vi "_RSA_PKCS1.vi"() -> ()   [LabVIEW 2023]
uses:
  <vilib>/addons/Tools/Unicode/UTF8 Tools.lvlib
panel:
  out "tick":u32
  in  "Tab Control":enum32{"密钥生成", "加密解密"}(tab)
  in  "生成秘钥":bool
  in  "填入密钥":bool
  out "公钥":string
  out "私钥":string
  out "?":string
  in  "密钥位数":string(combo)="308"
  in  "原文":string="Lorem ipsum dolor sit amet, consectetur adipisicing elit, sed do eiusmod tempor incididunt ut labore et dolore magna aliqua. Ut enim ad minim veniam, quis nostrud exercitation ullamco laboris nisi ut aliquip ex ea commodo consequat. Duis aute irure dolor in reprehenderit in voluptate velit esse cillum dolore eu fugiat nulla pariatur. Excepteur sint occaecat cupidatat non proident, sunt in culpa qui officia deserunt mollit anim id est laborum.\n"
  out "密文":string
  in  "密文":string="HCpIgJk/+R0CBhNWtByPKFZV9ITOXw7kY+R+gOsu/5SOpf9Kbk8F4EOCOOqLRaOCJf+GX3E+qD7oYj5SvAQCmhEU2YjpwG/wUmATbHKIMHQXZ3Rc/3We3BmbNaJrOw91EL7mVTCTQKMjuYVXiq0hajnJ+BwQXjJZfybkTRK94pGxM9G/5ZSGuP/ewRceAxQ0yhsyaCqbmHTiLNz3D6rYzJVMYsk9he5zXvHd+kh1cd+ASKWMB/Vgven+oDARy3ejDRk9U+cizFmNVrMUm57ClIMOirlQBShpa4uk4ZT/V0xm4sjeT+4QGanPMXhPoeHUftwo90kfVObeDCtFEM2rLgbRJHz2MoithAR2BuClGDqlx9vAYB7Ei8+WXeRKjW2AGi5rbdkcxlkdCeyQ6jcfV9paWfaTqELMHz1mj0miOK4jqfBWrivbPosi/fbzTefCRTtqdfDHCHDBJEmWznu712J68iJhvN7u1yrtBICKOHmNUei+4WFPm9bCTvQTIsQwz9hw1AqzWC64baBmIqTIvQTLyRJGjv1r6ERQIzWghyR0TXT+WTQWQxtIw4FetOOwLbTf1QXrQ6BoldZv3V28DkhC6P5vZM3x5ITuw08wj6Mt+oF41Nz+4hs4VaUNOiR2nf6cN2cOJvifRCPmeqlWFlGcHpX0+CvA145GZyN4+98="
  out "原文":string
  in  "加密":bool
  in  "解密":bool
  in  "公钥":string="-----BEGIN RSA PUBLIC KEY-----\nMIICCQKCAgBD33IPuq3zWwZXK/81Ebsg/7gVrV2vQ5o/0i/0ae8N/OOdEqVAupkM\nojXLqbPXJel1KlvTVMRJNtU45WlqnPDlWNInK6aqiPJHPAjOrX/lrrnaPksvRA2r\nfRN8VgmVZeQdT85luT3FWqZP7G2fsZq5Tp2bcm7265mnbctFlmg7BziyM5KmA5Hy\noUOkXDm2nWWwvsrr9evwZDpZTrLF2RoEP3Kb4uRrzjIEhBZer7fuM/m/wE728WyT\nuenw88mhmYYKpUHQn67jfuxqHOeFkRH/ShbL569eOh3pl2tDGEa7UTFxu31HLwje\n0zU3s59TWHqb7uISH5Dk+EqhKb3JfnHh5DfCO8qg7fRxGCk7yR6wb7WOG7kLnXz0\nuDfnWafYPiBqjywEnYkp8haQVAZSHtmvHw+ssjSRFV1kE0oMMB35+VKw1jkcQIQT\nxs9diDMW0j5Hb+LM86E5JwR3tKEHr3HWgOBcZJZ0woZGJ+gmNJ42F7XYxaeobkSR\nSRrFbEucK+l4q4FpkgwVS8L9NbUsu2CclK+Z2OI44Q3p44VI7ph6nfZrrVR02sHo\n5rIES8rVwXDdT1ory/Dq3SCOIRL6QC5zh6NTgZSYzwH1Jh8ufi07N+JToR1gdpM5\nc5wTTrmpFF+Ujk8lPEx7yZcZDbm70+2b9mAL7h+/7wy6Ia2Zjx4kGQIDAQAB\n-----END RSA PUBLIC KEY-----"
  in  "私钥":string="-----BEGIN RSA PRIVATE KEY-----\nMIIJJQIBAAKCAgBD33IPuq3zWwZXK/81Ebsg/7gVrV2vQ5o/0i/0ae8N/OOdEqVA\nupkMojXLqbPXJel1KlvTVMRJNtU45WlqnPDlWNInK6aqiPJHPAjOrX/lrrnaPksv\nRA2rfRN8VgmVZeQdT85luT3FWqZP7G2fsZq5Tp2bcm7265mnbctFlmg7BziyM5Km\nA5HyoUOkXDm2nWWwvsrr9evwZDpZTrLF2RoEP3Kb4uRrzjIEhBZer7fuM/m/wE72\n8WyTuenw88mhmYYKpUHQn67jfuxqHOeFkRH/ShbL569eOh3pl2tDGEa7UTFxu31H\nLwje0zU3s59TWHqb7uISH5Dk+EqhKb3JfnHh5DfCO8qg7fRxGCk7yR6wb7WOG7kL\nnXz0uDfnWafYPiBqjywEnYkp8haQVAZSHtmvHw+ssjSRFV1kE0oMMB35+VKw1jkc\nQIQTxs9diDMW0j5Hb+LM86E5JwR3tKEHr3HWgOBcZJZ0woZGJ+gmNJ42F7XYxaeo\nbkSRSRrFbEucK+l4q4FpkgwVS8L9NbUsu2CclK+Z2OI44Q3p44VI7ph6nfZrrVR0\n2sHo5rIES8rVwXDdT1ory/Dq3SCOIRL6QC5zh6NTgZSYzwH1Jh8ufi07N+JToR1g\ndpM5c5wTTrmpFF+Ujk8lPEx7yZcZDbm70+2b9mAL7h+/7wy6Ia2Zjx4kGQIDAQAB\nAoICADB+cPeOEQVELxaPh+t5/LLKItPSJ5K3AXnCCqNeIQBkhJhQnyPNbtbY+wjF\n+ompO9GL70niUdBhzhy1xQj4kyG6wYRdKtrDuB9vZHeO/Ue0/HNTeNKPlBjH5+k5\na+WDhGXxBG4n2VutthB6w6SK+BqYcgGD1Ia1tPYse0T//v7V3Qttz8Sv3lJ2KGdB\nwbaZZPPQjhnjfq0mX445rX+w62bHknKQvVXNYG1blsQWVptqJXJ8y66itkoiVmTj\nOlgs4dmvU4Pk48cFg5MZjc4f5bT6Ualkoyb27TJeDrREnxztGR/CrvLyRys1yts+\nioK5P/kzx/Dc/uCqCmB1+3UA1Ao/ptmaV1ZDMoYMTlaXkqPap6WsDN/I8p7xmSw9\n2LtirL6zHXTw5lIfoW87+lCdM37QtRexYCZPZH0kaGTs+xGVBiCdAsPyPqkoiFpP\noKkx0GRHmaZ0zab2Id6l+SBifzEa/6IU/t94mbsDyK/eK9AZjZhLjLreZEZmQWci\n8/c9NKOItkxBf+mLdxZDqeCmYHV4PbojLpCxqD0ngNo/y5CkegvP/Maq+6zkQ/Ci\nSIjUFnALqJx+HXf1BE+Qbs5TGOWLrs1y4+w8S4OnJ6S7ueVI/DkLlDHcT5c5S+W8\n/3/T1C/vgiJCKcT46sQAsl4KKIy6vKpQxtoMMbxe7zxVDgqRAoIBAQFz+6P3Y0to\nWhyAtUCneU6J/CN/ysVUr9EvvO/2fFYDSTeM3b7O1wvbkTanDFON/kbaDLllMp5S\nfWmkyWXcgm8lQ/Y7qakM902OPZ0hHLRrVyA2UcommOxhFCi5UrLJVtNkvxn44jpy\n1J2b7Pwap+pispIXdFEJ4So0It7Oh7V/XcOP0t7n4zM1EZ1qjnX6YCi3JinrB/9t\nQhlDLypv8ONLHx1EjBsVj21fMg1hAk32Clv4eS+EcNq6iqkJSmBFpsrGEkppLy8L\npmu4Og0S1D632tEXDDNTOc8RqD1aHkAVMYnnCPTWgd8W2DrAVXOjUL9HZXH84exV\nFfBYZQdFdiylAoIBAC611+BcPkzHP1B4giNZux1KMM5xwsGczd9Uwdjqm1JoquNn\njA2VSJhvIIOkSxkN8hh/lUpUXhWM7HJ8M/1eWcgrBJyskBnKb64fHIetZ6Ry9urD\nW5XO2MRAEfgN42F1P/glfv5UAjL+5/PBR69ddEV9YW42dJNAhfaIouzkFdEBxbXC\nJEE+bzoW3NcFCNCOJV0u41HQ0lLwWPqTz9zIqkGT0tAb26exyqfo/qmyIBnTT+Cd\ncXr8GKDgJZGOpTg7K4hy/L2+OJiAd8Lem9wkiMb8IfDqAdR0o50QFDXu1D/10CgK\nvCMBIUMlUWkzf/q8b39H/SAPt6tfZjsiRcG6u2UCggEAQDS/KIRLD8f+A3lFn6Kg\nm9CZkAU/6k4unT7PbIwpjIemvvnHZYxYz51RAaRvB6NMN3bayUzjZvmesoLQwi8B\nYD1K0yGFvGczS8n2xTBfM+fl93pGmkLrChagsNxFX9tMwab6pKrny8pHKhLNsQwq\nuL552PKKylnDHxyluKBUA5f7mWeccgoVXKOduDa+xmiynmpH8fl/bSxrj90kRg4e\nLWlBdAN66U3IYxYQmR38tusy1MCWIxYXqvskEiZ0V5Fijq25ik5KoIgpL7NVblqU\nOMfcL047zbG8vB9994AhL4dNdkNlf2ELULYh7fDR9O6LFZe9BRk54bXXtmo5xxOO\nwQKCAQAihZrK4uHYdNnCa44i+kpkV1TC/yjlVzKAgG/UFXA988V41CqaT16b6mWp\nZV9rYPcwS/rWOIxgeQq3gjwaYgUQ/1olQRQvO4JWuf+n9uzGiYEb+M5TZdCnGoMt\nRXZrrPBeQbgd15DYh7R+XrbQUM2CHixH/E8kFWfs0Qc49Ul6c0jgEGAjKDWkRQlq\nkPn2yVesCt9OtHr9eU0JxPy3PEc4uDvyOuSYh7ozZuvwFwnKjHZYl4QrVO4O2Bpr\n/XT2niSKcBGDWncRnsDkcQnYJdhA2E9tckVv89SIXD3TrnOH4fC551UsucUPjyEg\nE0Pe2C2/cEEP1Q31xkgUJDxR9eRRAoIBAGHW55fOf4K0b9SMA4+qDjSTC8FR8wjk\npKOPGwTb0qDzi1GgoFkViyBNeXbi/XhGvSgxktHB5rLHua5RV2CZ4hskDZFzHo12\nLTsHepyafJDLLefxP3ZXSOxKygcnBthiVShdR+Psk1xfljAWSxNTvHzhxIuzYCIq\nHgDA9mN/Ox47I3IktFOWXFYLp886eG4WXVYBW8DJ1ylreMCVZp2/R+ut25bnVfXS\n2DHVDJ325mwEP9aRwGh+KpbcA81X6KkZYtDIHzKOYRyp3exx05dFTQCceyXBOCHm\noG/bIfyOu/fk8RTQh3IRaIlvUEtZq5R5FmaHW/MMpnYutrLj1o00RUQ=\n-----END RSA PRIVATE KEY-----"
  in  "填入密文":bool
  out "加解密提示":string
  in  "填入密钥":bool
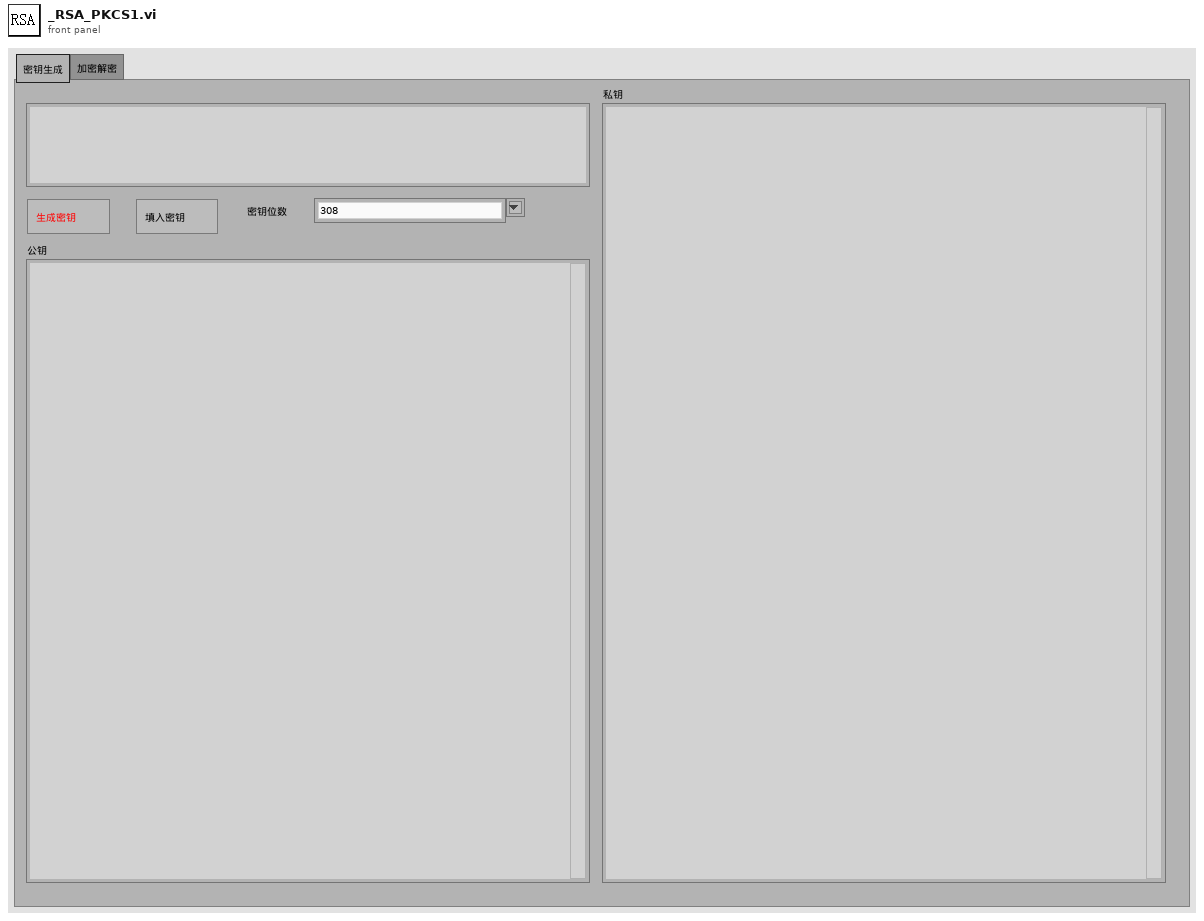
[diagram p1: front panel]
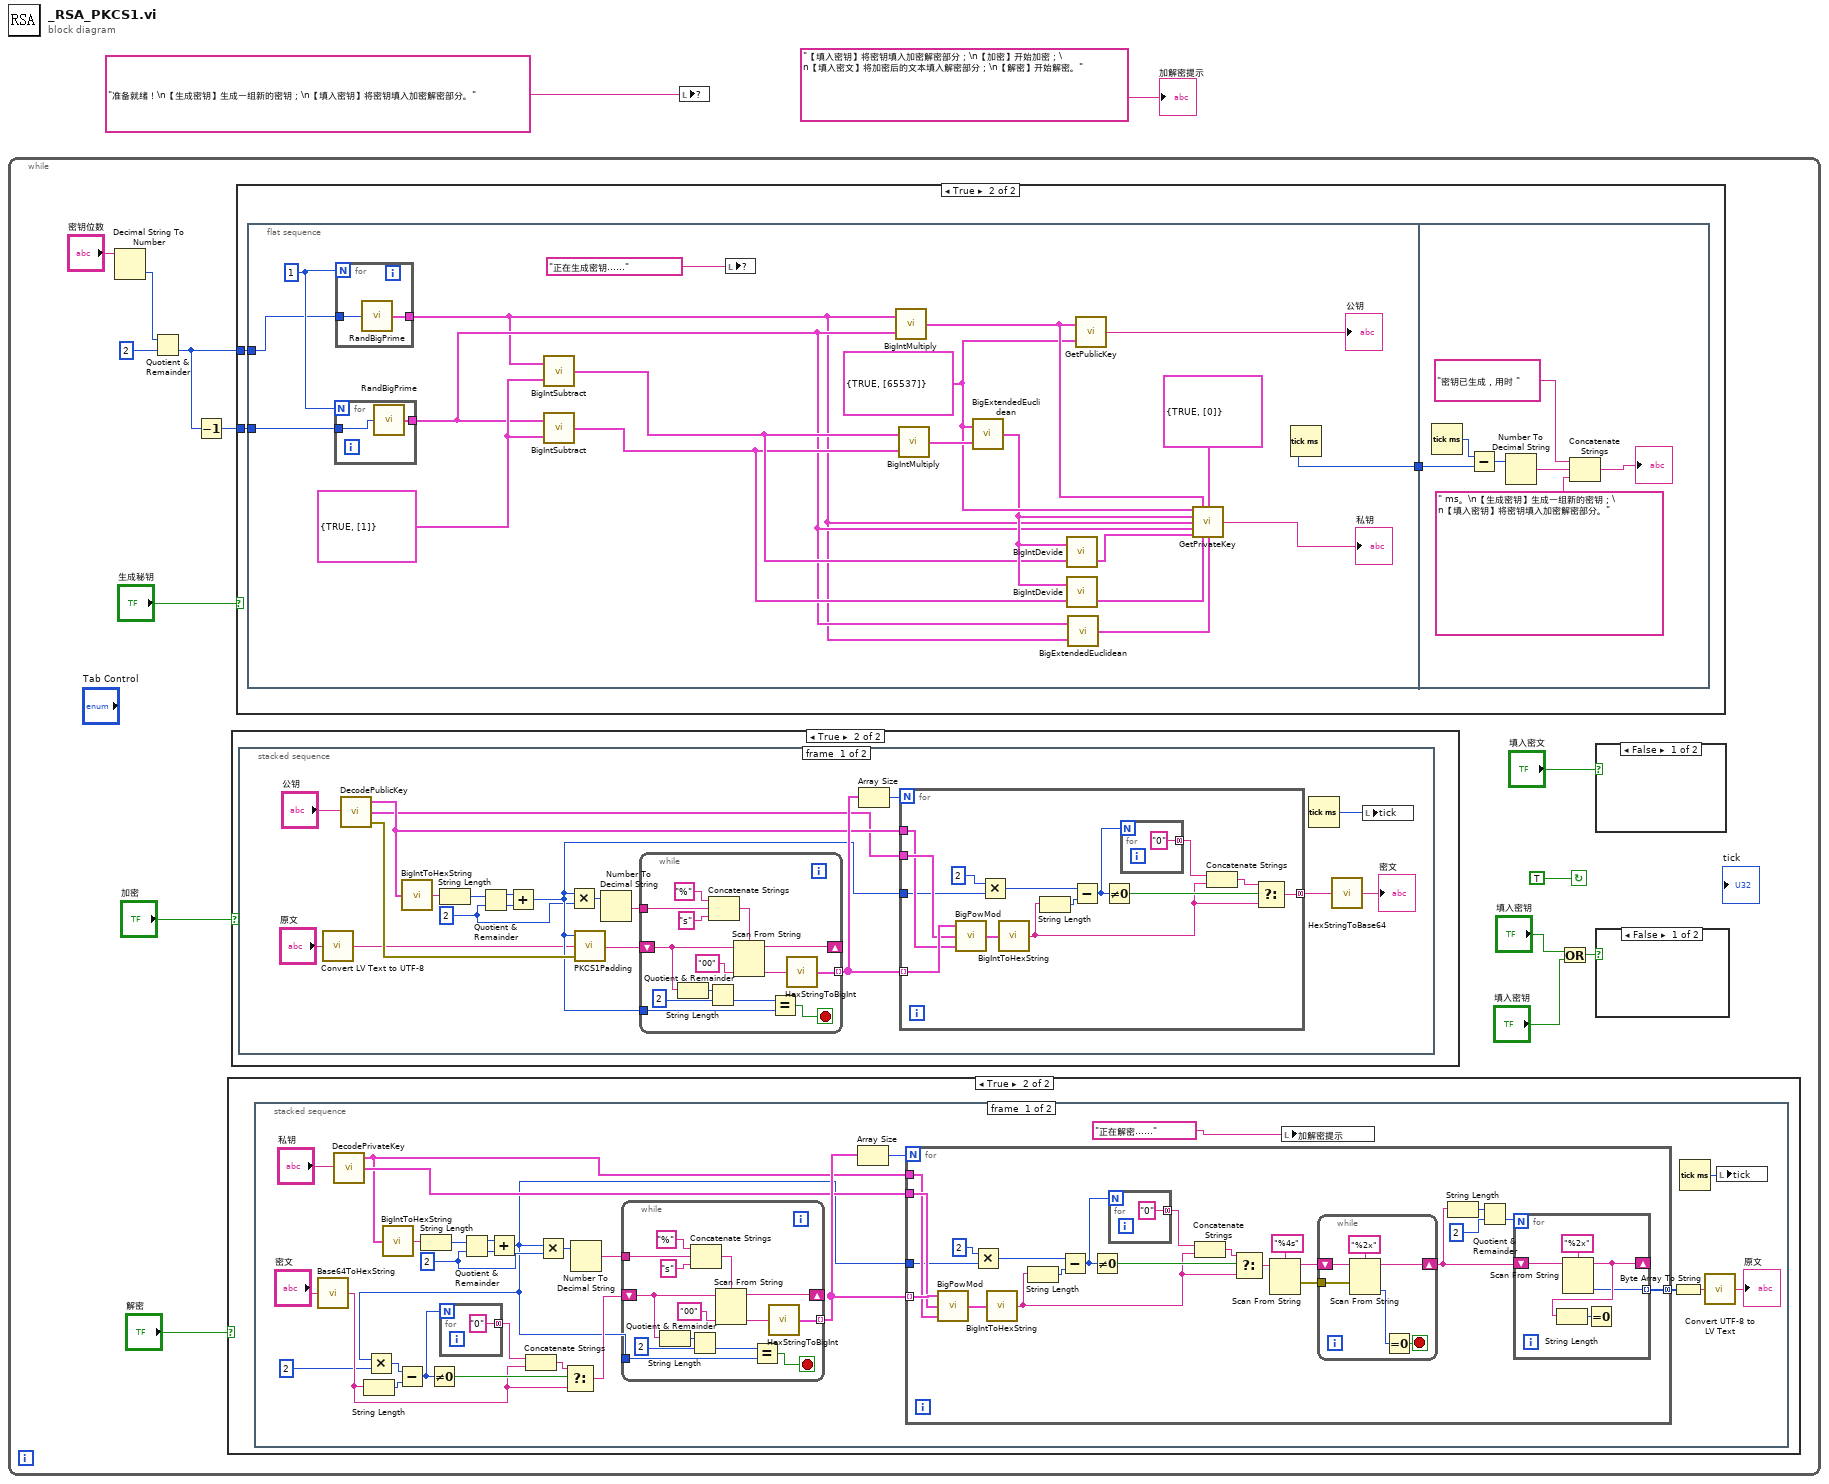
[diagram p0: block diagram]
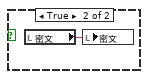
[diagram p2: hidden frame]
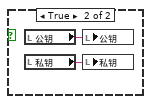
[diagram p3: hidden frame]
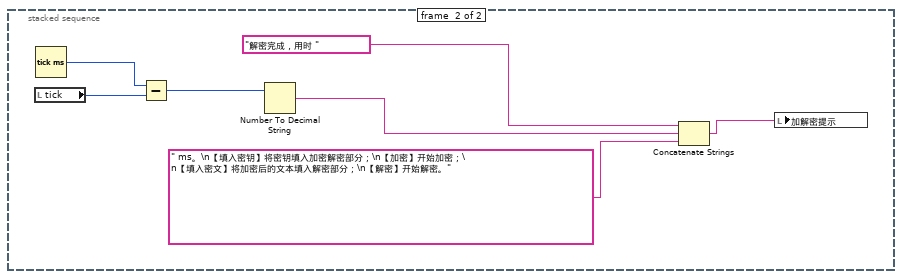
[diagram p5: hidden frame]
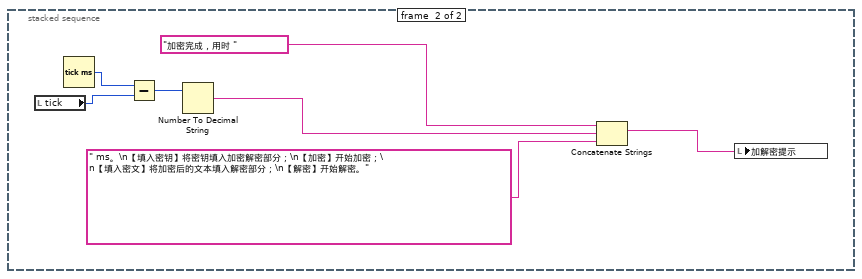
[diagram p7: hidden frame]
diagram:
  n1 = while {
    stop <- TRUE continue-if-true
    n2 = Decimal String To Number(string="密钥位数") -> (number=w8:i32)  [unwired: 2 in, 1 out]
    n3 = Quotient & Remainder(x=w8, y=2) -> (floor(x/y)=w7:i32)  [unwired: 1 out]
    n4 = Decrement(x=w7) -> (x-1=w6:i32)
    n5 = case shown="True" "解密" {
      frame False {
      }
      frame True {
        n6 = stacked-sequence {
          frame #0 {
            w41 = 2
            n7 = call "Base64ToHexString.vi"("BASE64 string"="密文") -> ("Hex"=w24:string)
            n8 = call "DecodePrivateKey.vi"("Private Key"="私钥") -> ("d"=w35:cluster{"P/N":bool, "Array":u64[]}, "n"=w34:cluster{"P/N":bool, "Array":u64[]})  [unwired: 2 in, 1 out]
            n9 = String Length(string=w24) -> (length=w30:i32)
            n10 = call "BigIntToHexString.vi"("a"=w34) -> ("Hex string"=w45:string)
            n11 = String Length(string=w45) -> (length=w44:i32)
            n12 = Quotient & Remainder(x=w44, y=w41) -> (x-y*floor(x/y)=w43:i32, floor(x/y)=w42:i32)
            n13 = Add(x=w43, y=w42) -> (x+y=w21:i32)
            n14 = Multiply(x=w21, y=2) -> (x*y=w22:i32)
            n15 = Subtract(x=w22, y=w30) -> (x-y=w28:i32)
            n16 = Not Equal To 0?(x=w28) -> (x != 0?=w29:bool)
            n17 = for {
              N: w28 -> [_]
              tunnel: ["0"] -> w27 mode=concatenating
            }
            n18 = Concatenate Strings(w27, w24) -> (w26:string)
            n19 = Multiply(x=w21, y=w41) -> (x*y=w40:i32)
            n20 = Select(t=w26, s=w29, f=w24) -> (s? t:f=w25:string)
            n21 = Number To Decimal String(number=w40) -> (decimal integer string=w39:string)  [unwired: 1 in]
            n22 = while {
              tunnel: w39 -> [w94]
              tunnel: w21 -> [w89]
              shift-right: [w86] -> _
              shift-left: w25 -> [w88]
              tunnel: [w85] -> w36 mode=indexing
              stop <- w87 stop-if-true
              n23 = String Length(string=w88) -> (length=w83:i32)
              n24 = Quotient & Remainder(x=w83, y=2) -> (floor(x/y)=w84:i32)  [unwired: 1 out]
              n25 = Concatenate Strings("%", w94, "s") -> (w92:string)
              n26 = Scan From String(format string=w92, input string=w88, default 1="00") -> (remaining string=w86:string, output 1=w90:string)  [unwired: 2 in, 2 out]
              n27 = Equal?(x=w84, y=w89) -> (x = y?=w87:bool)
              n28 = call "HexStringToBigInt.vi"("String (hex)"=w90) -> ("Int"=w85:cluster{"P/N":bool, "Array":u64[]})
            }
            n29 = Array Size(array=w36) -> (size(s)=w37:i32)
            n30 = for {
              N: w37 -> [_]
              tunnel: w36 -> [w69] mode=indexing
              tunnel: w35 -> [w68]
              tunnel: w34 -> [w67]
              tunnel: w21 -> [w54]
              tunnel: [w52] -> w33 mode=concatenating
              n31 = call "BigPowMod.vi"("c"=w67, "b"=w68, "a"=w69) -> ("a ^ b mod c"=w60:cluster{"Boolean":bool, "Array":u64[]})
              n32 = Multiply(x=2, y=w54) -> (x*y=w58:i32)
              n33 = call "BigIntToHexString.vi"("a"=w60) -> ("Hex string"=w62:string)
              n34 = String Length(string=w62) -> (length=w66:i32)
              n35 = Subtract(x=w58, y=w66) -> (x-y=w64:i32)
              n36 = Not Equal To 0?(x=w64) -> (x != 0?=w65:bool)
              n37 = for {
                N: w64 -> [_]
                tunnel: ["0"] -> w63 mode=concatenating
              }
              n38 = Concatenate Strings(w63, w62) -> (w61:string)
              n39 = Select(t=w61, s=w65, f=w62) -> (s? t:f=w57:string)
              n40 = Scan From String(format string="%4s", input string=w57) -> (remaining string=w53:string, error out=w55:errorcluster)  [unwired: 4 in, 1 out]
              n41 = while {
                tunnel: w55 -> [w80]
                shift-right: [w75] -> w51
                shift-left: w53 -> [w76]
                stop <- w77 stop-if-true
                n42 = Scan From String(format string="%2x", input string=w76, error in=w80) -> (remaining string=w75:string, output 1=w78:u32)  [unwired: 2 in, 2 out]
                n43 = Equal To 0?(x=w78) -> (x = 0?=w77:bool)
              }
              n44 = String Length(string=w51) -> (length=w49:i32)
              n45 = Quotient & Remainder(x=w49, y=2) -> (floor(x/y)=w50:i32)  [unwired: 1 out]
              n46 = for {
                N: w50 -> [_]
                shift-right: [w72] -> _
                shift-left: w51 -> [w73]
                tunnel: [w70] -> w52 mode=indexing
                n47 = Scan From String(format string="%2x", input string=w73) -> (remaining string=w72:string, output 1=w70:u32)  [unwired: 3 in, 2 out]
                n48 = String Length(string=w72) -> (length=w71:i32)
                n49 = Equal To 0?(x=w71) -> ()  [unwired: 1 out]
              }
            }
            n50 = local write "加解密提示"("正在解密……") -> ()
            n51 = Byte Array To String(unsigned byte array=w33) -> (string=w32:string)
            n52 = Tick Count (ms)() -> (millisecond timer value=w31:u32)
            n53 = call <vilib>:"Convert UTF-8 to LV Text.vi"("UTF-8 Text"=w32) -> ("LV Text"=→"原文":string)  [unwired: 13 in, 1 out]
            n54 = local write "tick"(w31) -> ()
          }
          frame #1 {
            n55 = local read "tick"() -> (w96:u32)
            n56 = Tick Count (ms)() -> (millisecond timer value=w97:u32)
            n57 = Subtract(x=w97, y=w96) -> (x-y=w102:u32)
            n58 = Number To Decimal String(number=w102) -> (decimal integer string=w100:string)  [unwired: 1 in]
            n59 = Concatenate Strings("解密完成，用时 ", w100, " ms。\n【填入密钥】将密钥填入加密解密部分；\n【加密】开始加密；\n【填入密文】将加密后的文本填入解密部分；\n【解密】开始解密。") -> (w98:string)
            n60 = local write "加解密提示"(w98) -> ()
          }
        }
      }
    }
    n61 = case shown="True" "加密" {
      frame False {
      }
      frame True {
        n62 = stacked-sequence {
          frame #0 {
            w105 = 2
            n63 = call <vilib>:"Convert LV Text to UTF-8.vi"("LV Text"="原文") -> ("UTF-8 Text"=w103:string)  [unwired: 13 in, 1 out]
            n64 = call "DecodePublicKey.vi"("Public Key"="公钥") -> ("error out"=w116:errorcluster, "e"=w110:cluster{"P/N":bool, "Array":u64[]}, "n"=w111:cluster{"P/N":bool, "Array":u64[]})  [unwired: 2 in]
            n65 = call "BigIntToHexString.vi"("a"=w111) -> ("Hex string"=w120:string)
            n66 = String Length(string=w120) -> (length=w119:i32)
            n67 = Quotient & Remainder(x=w119, y=w105) -> (x-y*floor(x/y)=w118:i32, floor(x/y)=w117:i32)
            n68 = Add(x=w118, y=w117) -> (x+y=w109:i32)
            n69 = Multiply(x=w109, y=w105) -> (x*y=w106:i32)
            n70 = call "PKCS1Padding.vi"("error in (no error)"=w116, "Message"=w103, "Length"=w109) -> ("Hex (After Padding)"=w115:string)  [unwired: 1 in, 1 out]
            n71 = Number To Decimal String(number=w106) -> (decimal integer string=w114:string)  [unwired: 1 in]
            n72 = while {
              tunnel: w114 -> [w150]
              tunnel: w109 -> [w145]
              shift-right: [w142] -> _
              shift-left: w115 -> [w144]
              tunnel: [w141] -> w112 mode=indexing
              stop <- w143 stop-if-true
              n73 = String Length(string=w144) -> (length=w139:i32)
              n74 = Quotient & Remainder(x=w139, y=2) -> (floor(x/y)=w140:i32)  [unwired: 1 out]
              n75 = Concatenate Strings("%", w150, "s") -> (w148:string)
              n76 = Scan From String(format string=w148, input string=w144, default 1="00") -> (remaining string=w142:string, output 1=w146:string)  [unwired: 2 in, 2 out]
              n77 = Equal?(x=w140, y=w145) -> (x = y?=w143:bool)
              n78 = call "HexStringToBigInt.vi"("String (hex)"=w146) -> ("Int"=w141:cluster{"P/N":bool, "Array":u64[]})
            }
            n79 = Array Size(array=w112) -> (size(s)=w113:i32)
            n80 = for {
              N: w113 -> [_]
              tunnel: w112 -> [w136] mode=indexing
              tunnel: w111 -> [w134]
              tunnel: w110 -> [w135]
              tunnel: w109 -> [w125]
              tunnel: [w129] -> w107 mode=concatenating
              n81 = call "BigPowMod.vi"("c"=w134, "b"=w135, "a"=w136) -> ("a ^ b mod c"=w133:cluster{"Boolean":bool, "Array":u64[]})
              n82 = Multiply(x=2, y=w125) -> (x*y=w127:i32)
              n83 = call "BigIntToHexString.vi"("a"=w133) -> ("Hex string"=w124:string)
              n84 = String Length(string=w124) -> (length=w132:i32)
              n85 = Subtract(x=w127, y=w132) -> (x-y=w130:i32)
              n86 = Not Equal To 0?(x=w130) -> (x != 0?=w131:bool)
              n87 = for {
                N: w130 -> [_]
                tunnel: ["0"] -> w128 mode=concatenating
              }
              n88 = Concatenate Strings(w128, w124) -> (w123:string)
              n89 = Select(t=w123, s=w131, f=w124) -> (s? t:f=w129:string)
            }
            n90 = Tick Count (ms)() -> (millisecond timer value=w104:u32)
            n91 = call "HexStringToBase64.vi"("Hex"=w107) -> ("BASE64 string"=→"密文":string)
            n92 = local write "tick"(w104) -> ()
          }
          frame #1 {
            n93 = local read "tick"() -> (w152:u32)
            n94 = Tick Count (ms)() -> (millisecond timer value=w153:u32)
            n95 = Subtract(x=w153, y=w152) -> (x-y=w158:u32)
            n96 = Number To Decimal String(number=w158) -> (decimal integer string=w156:string)  [unwired: 1 in]
            n97 = Concatenate Strings("加密完成，用时 ", w156, " ms。\n【填入密钥】将密钥填入加密解密部分；\n【加密】开始加密；\n【填入密文】将加密后的文本填入解密部分；\n【解密】开始解密。") -> (w154:string)
            n98 = local write "加解密提示"(w154) -> ()
          }
        }
      }
    }
    n99 = case shown="True" "生成秘钥" {
      tunnel: w7 -> [_ w159]
      tunnel: w6 -> [_ w160]
      frame False {
      }
      frame True {
        n100 = flat-sequence {
          tunnel: [w180] -> w161
          tunnel: w159 -> [w177]
          tunnel: w160 -> [w176]
          tunnel: w161 -> [w191]
          frame #0 {
            w170 = cluster{bool, u64[]} {TRUE, [65537]}
            w179 = 1
            w181 = cluster{bool, u64[]} {TRUE, [1]}
            n101 = for {
              N: w179 -> [_]
              tunnel: [w183] -> w164
              tunnel: w176 -> [w182]
              n102 = call "RandBigPrime.vi"("Numeric"=w182) -> ("Random Prime (1e18)"=w183:cluster{"Boolean":bool, "Array":u64[]})
            }
            n103 = for {
              N: w179 -> [_]
              tunnel: [w185] -> w163
              tunnel: w177 -> [w184]
              n104 = call "RandBigPrime.vi"("Numeric"=w184) -> ("Random Prime (1e18)"=w185:cluster{"Boolean":bool, "Array":u64[]})
            }
            n105 = call "BigIntSubtract.vi"("b"=w181, "a"=w163) -> ("a - b"=w168:cluster{"Boolean":bool, "Array":u64[]})
            n106 = call "BigIntSubtract.vi"("b"=w181, "a"=w164) -> ("a - b"=w167:cluster{"Boolean":bool, "Array":u64[]})
            n107 = local write item#13("正在生成密钥……") -> ()
            n108 = call "BigIntMultiply.vi"("b"=w164, "a"=w163) -> ("a * b"=w171:cluster{"Boolean":bool, "Array":u64[]})
            n109 = call "BigIntMultiply.vi"("b"=w167, "a"=w168) -> ("a * b"=w175:cluster{"Boolean":bool, "Array":u64[]})
            n110 = call "BigExtendedEuclidean.vi"("b"=w175, "a"=w170) -> ("c (ac mod(b) = 1)"=w169:cluster{"Boolean":bool, "Array":u64[]})
            n111 = call "BigIntDevide.vi"("b"=w168, "a"=w169) -> ("a % b"=w166:cluster{"Boolean":bool, "Array":u64[]})  [unwired: 1 out]
            n112 = call "BigIntDevide.vi"("b"=w167, "a"=w169) -> ("a % b"=w165:cluster{"Boolean":bool, "Array":u64[]})  [unwired: 1 out]
            n113 = call "BigExtendedEuclidean.vi"("b"=w163, "a"=w164) -> ("c (ac mod(b) = 1)"=w162:cluster{"Boolean":bool, "Array":u64[]})
            n114 = call "GetPublicKey.vi"("e"=w170, "n"=w171) -> ("Public Key"=→"公钥":string)
            n115 = call "GetPrivateKey.vi"("e"=w170, "n"=w171, "Version"=cluster{bool, u64[]} {TRUE, [0]}, "d"=w169, "p"=w163, "q"=w164, "d mod(p - 1)"=w166, "d mod(q - 1)"=w165, "q^-1 mod(p)"=w162) -> ("Public Key"=→"私钥":string)  [unwired: 6 in]
            n116 = Tick Count (ms)() -> (millisecond timer value=w180:u32)
          }
          frame #1 {
            n117 = Tick Count (ms)() -> (millisecond timer value=w192:u32)
            n118 = Subtract(x=w192, y=w191) -> (x-y=w190:u32)
            n119 = Number To Decimal String(number=w190) -> (decimal integer string=w188:string)  [unwired: 1 in]
            n120 = Concatenate Strings("密钥已生成，用时 ", w188, " ms。\n【生成密钥】生成一组新的密钥；\n【填入密钥】将密钥填入加密解密部分。") -> (→"?":string)
          }
        }
      }
    }
    n121 = Or(x="填入密钥", y="填入密钥") -> (x .or. y?=w5:bool)
    n122 = case shown="False" "填入密文" {
      frame False {
      }
      frame True {
        n123 = local read "密文"() -> (w16:string)
        n124 = local write "密文"(w16) -> ()
      }
    }
    n125 = case shown="False" w5 {
      frame False {
      }
      frame True {
        n126 = local read "公钥"() -> (w18:string)
        n127 = local read "私钥"() -> (w17:string)
        n128 = local write "公钥"(w18) -> ()
        n129 = local write "私钥"(w17) -> ()
      }
    }
  }
  n130 = local write item#13("准备就绪！\n【生成密钥】生成一组新的密钥；\n【填入密钥】将密钥填入加密解密部分。") -> ()
  "加解密提示" <- "【填入密钥】将密钥填入加密解密部分；\n【加密】开始加密；\n【填入密文】将加密后的文本填入解密部分；\n【解密】开始解密。"
